vi "Init_tree.vi"(7 "Notes":string[](array[string]), 10 "First Call?: T/F":bool, 11 "TreeControl in":refnum<vi>) -> ()   [LabVIEW 2019, in "Visual.xctl"]
uses:
  Visual.xctl
  <vilib>/Utility/miscctls.llb/LVRowAndColumnTypeDef.ctl
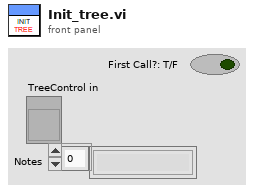
[diagram p1: front panel]
types:
  T1 = typedef "LVRowAndColumnTypeDef.ctl" = cluster{"Row":i32, "Column":i32}
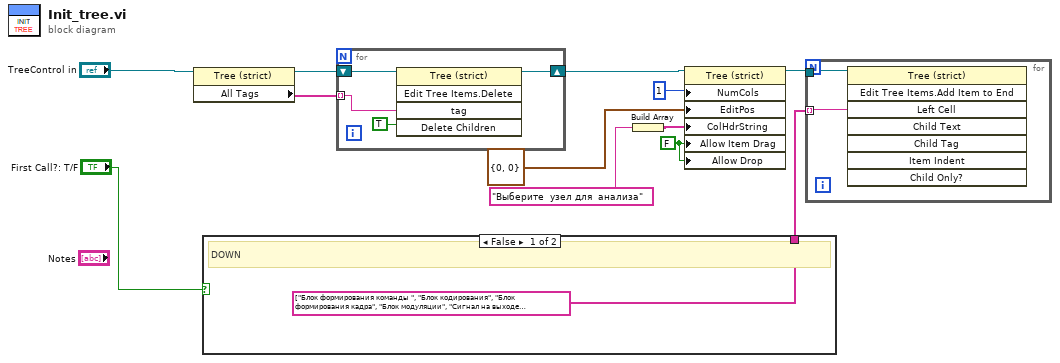
[diagram p0: block diagram]
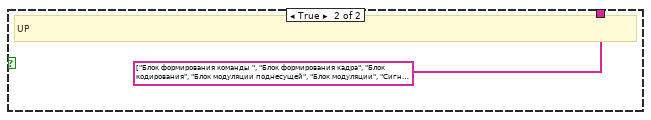
[diagram p2: hidden frame]
diagram:
  w11 = FALSE ("Drag/Drop:Allow Dragging")
  n1 = property class="Tree (strict)"(reference="TreeControl in") -> (reference out=w4:refnum<vi>, "All Tags"=w3:string[])  [unwired: 1 in, 1 out]
  n2 = case shown="False" "First Call?: T/F" {
    tunnel: [string[] ["Блок формирования команды ", "Блок кодирования", "Блок формирования кадра", "Блок модуляции", "Сигнал на выходе считывателя", "Сигнал с шумом", "Сигнал на входе метки", "Блок демодуляции", "Блок проверки кадра", "Блок декодирования"] ("Column Header Strings[]") string[] ["Блок формирования команды ", "Блок формирования кадра", "Блок кодирования", "Блок модуляции поднесущей", "Блок модуляции", "Сигнал на выходе метки", "Сигнал с шумом", "Сигнал на входе считывателя", "Блок демодуляции", "Блок демодуляции поднесущей", "Блок декодирования", "Блок проверки кадра"] ("Column Header Strings[]")] -> w10
    frame False {
      # "DOWN"
    }
    frame True {
      # "UP"
    }
  }
  n3 = for {
    shift-right: [w18] -> w2
    shift-left: w4 -> [w16]
    tunnel: w3 -> [w15] mode=indexing
    n4 = invoke class="Tree (strict)" method="Edit Tree Items.Delete"(reference=w16, "tag"=w15, "Delete Children"=TRUE ("Delete Children?")) -> (reference out=w18:refnum<vi>)  [unwired: 2 in, 4 out]
  }
  n5 = Build Array("Выберите  узел для  анализа") -> (w9:string[])
  n6 = property on="Property Node" class="Tree (strict)"(reference=w2, "NumCols"=u32 1 ("Number of Columns"), "EditPos"=T1 {"Row"=0, "Column"=0} ("Edit Position"), "ColHdrString"=w9, "Allow Item Drag"=w11, "Allow Drop"=w11) -> (reference out=w7:refnum<vi>)  [unwired: 1 in, 1 out]
  n7 = for {
    tunnel: w7 -> [w20]
    tunnel: w10 -> [w19] mode=indexing
    n8 = invoke class="Tree (strict)" method="Edit Tree Items.Add Item to End"(reference=w20, "Left Cell"=w19) -> ()  [unwired: 6 in, 8 out]
  }
